vi "Single Motor Init.vi"(0 "Motor In":T1={"Motor1"={"DeviceStatus"={"status"=FALSE, "code"=0, "source"=""}, "Type"=enum."PWM", "PWM"={"PWM Channel"=enum."Invalid", "DeadBand"={"Name"="", "maxPositivePwm"=0, "minPositivePwm"=0, "centerPwm"=0, "maxNegativePwm"=0, "minNegativePwm"=0, "angularRange"=0}}, "CAN"={"Device Number"=0, "Control Mode"=enum."Percent VBus", "Semaphore"=refnum, "Max Vout"=12.0, "TalonSRX Control Mode"=enum."Percent VBus"}, "Invert"=FALSE}, "Last Motor Power"=0.0}, 1 "PWM Channel":T4, 5 "CAN Id":u8, 7 "Use Can":bool, 9 "Invert (default false)":bool, 11 "error in":errorcluster) -> (4 "Motor Out":T1={"Motor1"={"DeviceStatus"={"status"=FALSE, "code"=0, "source"=""}, "Type"=enum."PWM", "PWM"={"PWM Channel"=enum."Invalid", "DeadBand"={"Name"="", "maxPositivePwm"=0, "minPositivePwm"=0, "centerPwm"=0, "maxNegativePwm"=0, "minNegativePwm"=0, "angularRange"=0}}, "CAN"={"Device Number"=0, "Control Mode"=enum."Percent VBus", "Semaphore"=refnum, "Max Vout"=12.0, "TalonSRX Control Mode"=enum."Percent VBus"}, "Invert"=FALSE}, "Last Motor Power"=0.0}, 15 "error out":errorcluster)   [LabVIEW 2015]
uses:
  <vilib>/Rock Robotics/SystemInterfaces/DIO/FPGA_DIOPWMChannel.ctl
  Motor Typedef.ctl
  <vilib>/Rock Robotics/WPI/MotorControl/WPI_MotorControlDeviceRef.ctl
  <vilib>/Rock Robotics/WPI/MotorControl/WPI_MotorControlType.ctl
  <vilib>/Rock Robotics/WPI/PWM/WPI_PWMDeadband.ctl
  <vilib>/Rock Robotics/WPI/CAN/Jaguar/SubVIs/WPI_CANJaguar_ControlMode.ctl
  <vilib>/Rock Robotics/WPI/CAN/TalonSRX/WPI_CANTalonSRX_APIControlMode.ctl
  Support/Global Objects.vi
  <vilib>/Rock Robotics/WPI/MotorControl/WPI_MotorControlOpenCANTalonSRX.vi
  <vilib>/Rock Robotics/WPI/MotorControl/WPI_MotorControlOpen VictorSP.vi
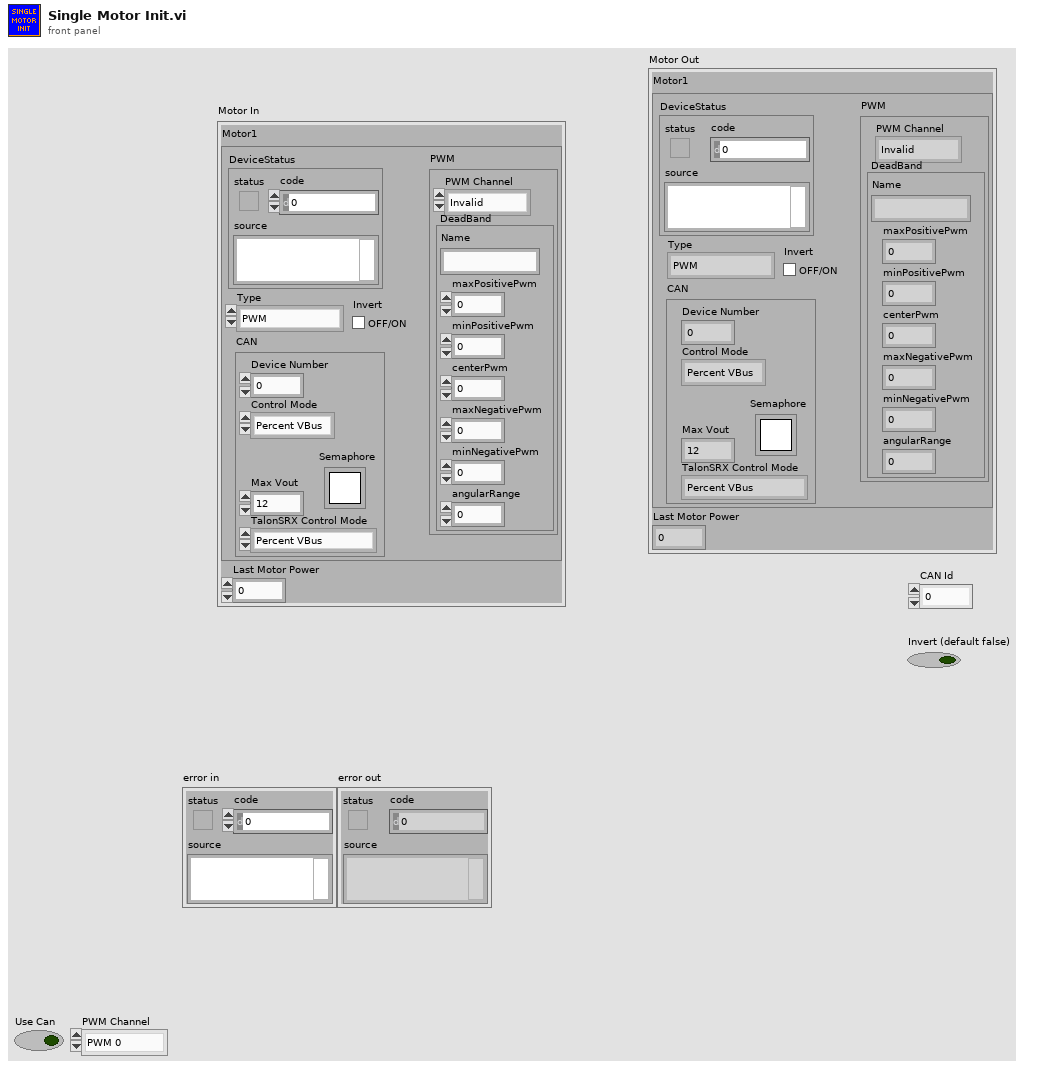
[diagram p1: front panel]
types:
  T1 = typedef "Motor Typedef.ctl" = cluster{"Motor1":T2, "Last Motor Power":dbl}
  T2 = typedef "WPI_MotorControlDeviceRef.ctl" = cluster{"DeviceStatus":errorcluster, "Type":T3, "PWM":cluster{"PWM Channel":T4, "DeadBand":T5}, "CAN":cluster{"Device Number":u8, "Control Mode":T6, "Semaphore":T7, "Max Vout":dbl, "TalonSRX Control Mode":T8}, "Invert":bool}
  T3 = typedef "WPI_MotorControlType.ctl" = enum16{"PWM", "CAN", "CANTalonSRX"}
  T4 = typedef "FPGA_DIOPWMChannel.ctl" = enum8{"PWM 0", "PWM 1", "PWM 2", "PWM 3", "PWM 4", "PWM 5", "PWM 6", "PWM 7", "PWM 8", "PWM 9", "PWM MXP 0", "PWM MXP 1", "PWM MXP 2", "PWM MXP 3", "PWM MXP 4", "PWM MXP 5", "PWM MXP 6", "PWM MXP 7", "PWM MXP 8", "PWM MXP 9", "Invalid"}
  T5 = typedef "WPI_PWMDeadband.ctl" = cluster{"Name":string, "maxPositivePwm":i32, "minPositivePwm":i32, "centerPwm":i32, "maxNegativePwm":i32, "minNegativePwm":i32, "angularRange":u16}
  T6 = typedef "WPI_CANJaguar_ControlMode.ctl" = enum8{"Percent VBus", "Current", "Speed", "Position", "Voltage"}
  T7 = typedef "Semaphore RefNum" = refnum<k1>
  T8 = typedef "WPI_CANTalonSRX_APIControlMode.ctl" = enum8{"Percent VBus", "Speed", "Position", "Slave", "Unchanged / Invalid", "Voltage Compensation", "Current", "Motion Profile"}
  T9 = typedef "Configuration.ctl" = cluster{"Throttle Dead Zone":dbl, "Throttle Ramp Rate":dbl, "Turn Dead Zone":dbl, "Auton":cluster{"Motion Plan P":dbl, "Motion Plan I":dbl, "Motion Plan D":dbl}, "Auto Upshift Enabled":bool, "Upshift Min Throttle":dbl, "Upshift Min Velocity":dbl, "Min time before upshift":dbl, "Shift Throttle Detent":u32, "Min time before downshift":dbl, "Turn PID":cluster{"Motion Plan P":dbl, "Motion Plan I":dbl, "Motion Plan D":dbl}, "Auto Coast Downshift":bool, "Downshift Coast Max Vel":dbl, "Downshift Coast Throttle Epsilon":dbl, "Left Motor Calibration":dbl, "Right Motor Calibration":dbl, "Tank Mode":bool, "Shooter PID":cluster{"Shooter  P":dbl, "Shooter  I":dbl, "Shooter  D":dbl}}
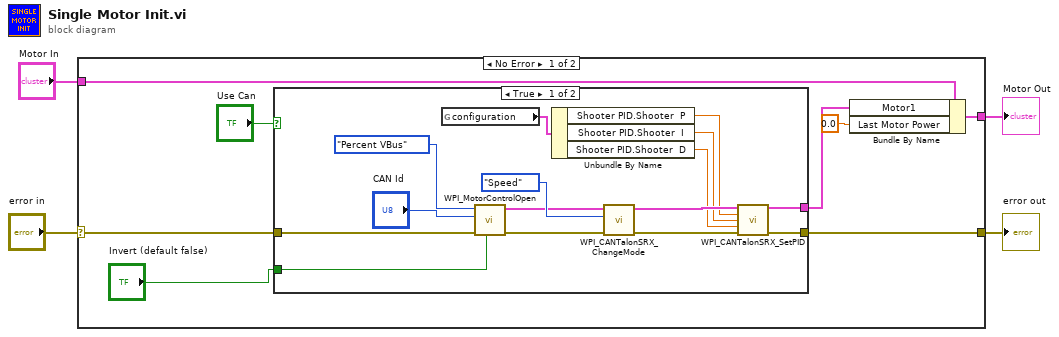
[diagram p0: block diagram]
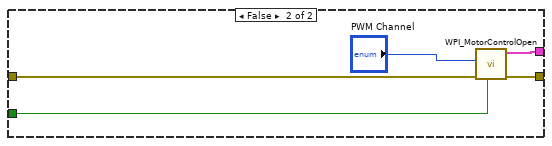
[diagram p2: hidden frame]
diagram:
  n1 = case shown="No Error" "error in" {
    selector: "error in" -> [w9 w33]
    tunnel: "Motor In" -> [w11 w34]
    tunnel: [w10 w34] -> w1
    tunnel: [w8 w33] -> w3
    frame No Error {
      n2 = case shown="True" "Use Can" {
        tunnel: [w18 w32] -> w12
        tunnel: w9 -> [w25 w31]
        tunnel: [w17 w28] -> w8
        tunnel: "Invert (default false)" -> [w24 w29]
        frame True {
          n3 = global read "Global Objects.vi" "configuration"() -> (w16:T9)
          n4 = call-poly <vilib>:"WPI_MotorControlOpen.vi"("Invert"=w24, "error in (no error)"=w25, "Device Number"="CAN Id", "Control Mode"=WPI_CANTalonSRX_APIControlMode."Percent VBus") -> ("error out"=w21:errorcluster, "MotorControlDeviceRef"=w22:T2)  [unwired: 6 in]
          n5 = Unbundle By Name(w16) -> ("Shooter PID.Shooter  P"=w15:dbl, "Shooter PID.Shooter  I"=w14:dbl, "Shooter PID.Shooter  D"=w13:dbl)
          n6 = call <vilib>:"WPI_CANTalonSRX_ChangeMode.vi"("error in (no error)"=w21, "Control Mode"=WPI_CANTalonSRX_APIControlMode."Speed", "CAN Talon SRX Ref"=w22) -> ("error out"=w20:errorcluster, "CAN Talon SRX Ref"=w19:T2)  [unwired: 7 in]
          n7 = call <vilib>:"WPI_CANTalonSRX_SetPID.vi"("CAN Talon SRX Ref"=w19, "P"=w15, "I"=w14, "D"=w13, "error in (no error)"=w20) -> ("CAN Talon SRX Ref"=w18:T2, "error out"=w17:errorcluster)  [unwired: 9 in]
        }
        frame False {
          n8 = call-poly <vilib>:"WPI_MotorControlOpen.vi"("Invert"=w29, "error in (no error)"=w31, "PWM Channel"="PWM Channel") -> ("error out"=w28:errorcluster, "MotorControlDeviceRef"=w32:T2)  [unwired: 7 in]
        }
      }
      n9 = Bundle By Name(cluster=w11, "Motor1"=w12, "Last Motor Power"=0.0) -> (w10:T1)
    }
    frame Error {
    }
  }
  "error out" <- w3
  "Motor Out" <- w1
